vi "Delay Generator SG08p.vi"() -> ()   [LabVIEW 2009, in "POLARIS BME DG.lvlib"]
uses:
  POLARIS BME DG.lvlib
  SubVI/Settings G08.ctl
  <vilib>/Utility/error.llb/DialogType.ctl
panel:
  in  "Settings":T1={"Channel A"={"Delay (µs)"=0.013000000000000001, "Pulse Width (µs)"=0.019, "Output Modulo"=1, "Output Offset"=0, "Go Signal"=16, "Polarity"=TRUE, "Terminate"=FALSE}, "Channel B"={"Delay (µs)"=0.032, "Pulse Width (µs)"=0.019, "Output Modulo"=1, "Output Offset"=0, "Go Signal"=16, "Polarity"=TRUE, "Terminate"=FALSE}, "Channel C"={"Delay (µs)"=0.0, "Pulse Width (µs)"=0.01, "Output Modulo"=1, "Output Offset"=0, "Go Signal"=16, "Polarity"=TRUE, "Terminate"=FALSE}, "Channel D"={"Delay (µs)"=0.01, "Pulse Width (µs)"=0.01, "Output Modulo"=1, "Output Offset"=0, "Go Signal"=16, "Polarity"=TRUE, "Terminate"=FALSE}, "Channel E"={"Delay (µs)"=0.0, "Pulse Width (µs)"=0.01, "Output Modulo"=1, "Output Offset"=0, "Go Signal"=16, "Polarity"=TRUE, "Terminate"=FALSE, "Disconnect"=FALSE, "Onto MsBus"=FALSE, "Input Positive"=TRUE}, "Channel F"={"Delay (µs)"=0.0, "Pulse Width (µs)"=0.01, "Output Modulo"=1, "Output Offset"=0, "Go Signal"=16, "Polarity"=TRUE, "Terminate"=FALSE, "Disconnect"=FALSE, "Onto MsBus"=FALSE, "Input Positive"=TRUE}, "Clock Enable"=TRUE, "Ocillator Divider"=2, "Trigger Divider"=1, "Trigger Multiplier"=4, "Clock Source"=3, "Trigger Terminate"=TRUE, "Gate Terminate"=TRUE, "Trigger Level"=0.2, "Gate Level"=0.0, "Gate Delay (µs)"=-1.0, "MS Bus"=1, "Internal Clock (µs)"=0.0083333, "Stop Trigger"=1, "Gate Divider"=0, "Force Trigger (µs)"=-1.0, "Step Back Time (µs)"=-1.0, "Burst Counter"=1, "Positive Gate"=TRUE, "Trigger Source"=TRUE, "Gate Type"=TRUE, "Synchronize Gate"=FALSE, "Trigger Slope"=TRUE, "Stop on Preset"=FALSE, "Reset When Done"=TRUE, "Trigger Enable"=TRUE, "Gate AB"=0, "Gate CD"=0, "Gate EF"=0} {"Gate EF" items=["Normal"=0, "EF_OR"=1048576, "EF_AND"=2097152, "EF_XOR"=3145728]; "Gate CD" items=["Normal"=0, "CD_OR"=262144, "CD_AND"=524288, "CD_XOR"=786432]; "Gate AB" items=["Normal"=0, "AB_OR"=65536, "AB_AND"=131072, "AB_XOR"=196608]; "Step Back Time (µs)" min=-1.0 format="%.6f"; "Force Trigger (µs)" min=-1.0 format="%.6f"; "Gate Delay (µs)" min=-1.0 format="%.6f"; "Internal Clock (µs)" min=0.0 format="%.6f"; "MS Bus" format="%04x" items=["Local Primary"=1, "Local Secondary"=2, "Local Force"=4, "Resynchronize"=8, "Master Primary"=16, "Master Secondary"=32, "Master Force"=64, "System Clock"=128, "Delay Clock"=256, "Inhibit Local"=512, "Start Local"=1024, "Start Bus"=2048, "Step Back Local"=4096, "Step Back Bus"=8192, "Enable From E"=65536, "Enable From F"=131072, "Enable From Bus"=262144]; "Gate Level" min=-2.5 max=2.5 format="%.3g"; "Trigger Level" min=-2.5 max=2.5 format="%.3f"; "Clock Source" items=["Internal Oscillator"=1, "External Trigger"=2, "Trigger & Oscillator"=3, "Master Slave Bus"=4]; "Trigger Multiplier" min=1; "Trigger Divider" min=1; "Ocillator Divider" min=1; "Channel F"."Go Signal" format="%04x" items=["Loc Prim"=1, "Loc Sec"=2, "Loc Force"=4, "Resynch"=8, "Mas Prim"=16, "Mas Sec"=32, "Mas Force"=64, "Sys Clock"=128, "Delay Clock"=256, "Inhibit Local"=512, "Start Local"=1024, "Start Bus"=2048, "Step Back Loc"=4096, "Step Back Bus"=8192, "From E"=65536, "From F"=131072, "From Bus"=262144]; "Channel F"."Pulse Width (µs)" min=0.0 max=8947840.0 format="%.6f"; "Channel F"."Delay (µs)" min=0.0 format="%.6f"; "Channel E"."Go Signal" format="%04x" items=["Loc Prim"=1, "Loc Sec"=2, "Loc Force"=4, "Resynch"=8, "Mas Prim"=16, "Mas Sec"=32, "Mas Force"=64, "Sys Clock"=128, "Delay Clock"=256, "Inhibit Local"=512, "Start Local"=1024, "Start Bus"=2048, "Step Back Loc"=4096, "Step Back Bus"=8192, "From E"=65536, "From F"=131072, "From Bus"=262144]; "Channel E"."Pulse Width (µs)" min=0.0 max=8947840.0 format="%.6f"; "Channel E"."Delay (µs)" min=0.0 format="%.6f"; "Channel D"."Go Signal" format="%04x" items=["Loc Prim"=1, "Loc Sec"=2, "Loc Force"=4, "Resynch"=8, "Mas Prim"=16, "Mas Sec"=32, "Mas Force"=64, "Sys Clock"=128, "Delay Clock"=256, "Inhibit Local"=512, "Start Local"=1024, "Start Bus"=2048, "Step Back Loc"=4096, "Step Back Bus"=8192, "From E"=65536, "From F"=131072, "From Bus"=262144]; "Channel D"."Pulse Width (µs)" min=0.0 max=8947840.0 format="%.6f"; "Channel D"."Delay (µs)" min=0.0 format="%.6f"; "Channel C"."Go Signal" format="%04x" items=["Loc Prim"=1, "Loc Sec"=2, "Loc Force"=4, "Resynch"=8, "Mas Prim"=16, "Mas Sec"=32, "Mas Force"=64, "Sys Clock"=128, "Delay Clock"=256, "Inhibit Local"=512, "Start Local"=1024, "Start Bus"=2048, "Step Back Loc"=4096, "Step Back Bus"=8192, "From E"=65536, "From F"=131072, "From Bus"=262144]; "Channel C"."Pulse Width (µs)" min=0.0 max=8947840.0 format="%.6f"; "Channel C"."Delay (µs)" min=0.0 format="%.6f"; "Channel B"."Go Signal" format="%04x" items=["Loc Prim"=1, "Loc Sec"=2, "Loc Force"=4, "Resynch"=8, "Mas Prim"=16, "Mas Sec"=32, "Mas Force"=64, "Sys Clock"=128, "Delay Clock"=256, "Inhibit Local"=512, "Start Local"=1024, "Start Bus"=2048, "Step Back Loc"=4096, "Step Back Bus"=8192, "From E"=65536, "From F"=131072, "From Bus"=262144]; "Channel B"."Pulse Width (µs)" min=0.0 max=8947840.0 format="%.6f"; "Channel B"."Delay (µs)" min=0.0 format="%.6f"; "Channel A"."Go Signal" format="%04x" items=["Loc Prim"=1, "Loc Sec"=2, "Loc Force"=4, "Resynch"=8, "Mas Prim"=16, "Mas Sec"=32, "Mas Force"=64, "Sys Clock"=128, "Delay Clock"=256, "Inhibit Local"=512, "Start Local"=1024, "Start Bus"=2048, "Step Back Loc"=4096, "Step Back Bus"=8192, "From E"=65536, "From F"=131072, "From Bus"=262144]; "Channel A"."Pulse Width (µs)" min=0.0 max=8947840.0 format="%.6f"; "Channel A"."Delay (µs)" min=0.0 format="%.6f"}
  in  "Exit":bool
  # "NOTICE -- YOU MUST LEAVE THIS NOTICE IN PLACE.  PER THE TERMS OF THE LICENSE BELOW, YOU MAY SUBLICENSE THIS SOFTWARE \nIN ANY WAY THAT DOES NOT CONFLICT WITH THIS LICENSE.\n\n### BSD License (http://www.opensource.org/licenses/bsd-license.php) Begin ###\n \nCopyright (c) 2011, Applied Energetics, http://www.appliedenergetics.com,\n                               Richard Schwerdtfeger, <rschwerdtfeger@appliedenergetics.com>\n\nAll rights reserved.\n\nRedistribution and use in source and binary forms, with or without modification, are permitted provided that the \nfollowing conditions are met:\n\n    * Redistributions of source code must retain the above copyright notice, this list of conditions and the following disclaimer.\n    * Redistributions in binary form must reproduce the above copyright notice, this list of conditions and the following disclaimer \n       in the documentation and/or other materials provided with the distribution.\n    * Neither the name of Richard Schwerdtfeger, Applied Energetics, Inc., nor the names of its contributors may be used to \n       endorse or promote products derived from this software without specific prior written permission.\n\nTHIS SOFTWARE IS PROVIDED BY THE COPYRIGHT HOLDERS AND CONTRIBUTORS \"AS IS\" AND ANY EXPRESS OR IMPLIED WARRANTIES, \nINCLUDING, BUT NOT LIMITED TO, THE IMPLIED WARRANTIES OF MERCHANTABILITY AND FITNESS FOR A PARTICULAR PURPOSE ARE \nDISCLAIMED. IN NO EVENT SHALL THE COPYRIGHT OWNER OR CONTRIBUTORS BE LIABLE FOR ANY DIRECT, INDIRECT, INCIDENTAL,\n SPECIAL, EXEMPLARY, OR CONSEQUENTIAL DAMAGES (INCLUDING, BUT NOT LIMITED TO, PROCUREMENT OF SUBSTITUTE GOODS OR \nSERVICES; LOSS OF USE, DATA, OR PROFITS; OR BUSINESS INTERRUPTION) HOWEVER CAUSED AND ON ANY THEORY OF LIABILITY, \nWHETHER IN CONTRACT, STRICT LIABILITY, OR TORT (INCLUDING NEGLIGENCE OR OTHERWISE) ARISING IN ANY WAY OUT OF THE USE \nOF THIS SOFTWARE, EVEN IF ADVISED OF THE POSSIBILITY OF SUCH DAMAGE.\n\n### BSD License End ###"
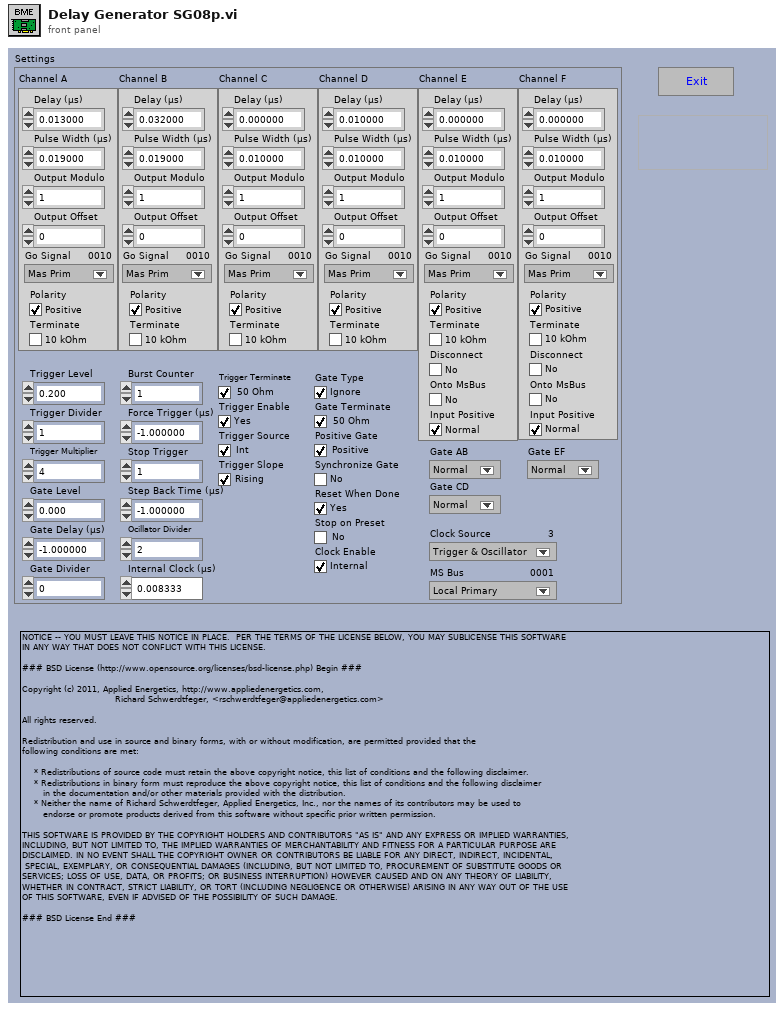
[diagram p1: front panel]
types:
  T1 = typedef "POLARIS BME DG.lvlib/Settings G08.ctl" = cluster{"Channel A":cluster{"Delay (µs)":dbl, "Pulse Width (µs)":dbl, "Output Modulo":u32, "Output Offset":u32, "Go Signal":u32, "Polarity":bool, "Terminate":bool}, "Channel B":cluster{"Delay (µs)":dbl, "Pulse Width (µs)":dbl, "Output Modulo":u32, "Output Offset":u32, "Go Signal":u32, "Polarity":bool, "Terminate":bool}, "Channel C":cluster{"Delay (µs)":dbl, "Pulse Width (µs)":dbl, "Output Modulo":u32, "Output Offset":u32, "Go Signal":u32, "Polarity":bool, "Terminate":bool}, "Channel D":cluster{"Delay (µs)":dbl, "Pulse Width (µs)":dbl, "Output Modulo":u32, "Output Offset":u32, "Go Signal":u32, "Polarity":bool, "Terminate":bool}, "Channel E":cluster{"Delay (µs)":dbl, "Pulse Width (µs)":dbl, "Output Modulo":u32, "Output Offset":u32, "Go Signal":u32, "Polarity":bool, "Terminate":bool, "Disconnect":bool, "Onto MsBus":bool, "Input Positive":bool}, "Channel F":cluster{"Delay (µs)":dbl, "Pulse Width (µs)":dbl, "Output Modulo":u32, "Output Offset":u32, "Go Signal":u32, "Polarity":bool, "Terminate":bool, "Disconnect":bool, "Onto MsBus":bool, "Input Positive":bool}, "Clock Enable":bool, "Ocillator Divider":u32, "Trigger Divider":u32, "Trigger Multiplier":u32, "Clock Source":u32, "Trigger Terminate":bool, "Gate Terminate":bool, "Trigger Level":dbl, "Gate Level":dbl, "Gate Delay (µs)":dbl, "MS Bus":u32, "Internal Clock (µs)":dbl, "Stop Trigger":u32, "Gate Divider":u32, "Force Trigger (µs)":dbl, "Step Back Time (µs)":dbl, "Burst Counter":u32, "Positive Gate":bool, "Trigger Source":bool, "Gate Type":bool, "Synchronize Gate":bool, "Trigger Slope":bool, "Stop on Preset":bool, "Reset When Done":bool, "Trigger Enable":bool, "Gate AB":u32, "Gate CD":u32, "Gate EF":u32}
  T2 = typedef "DialogType.ctl" = u16
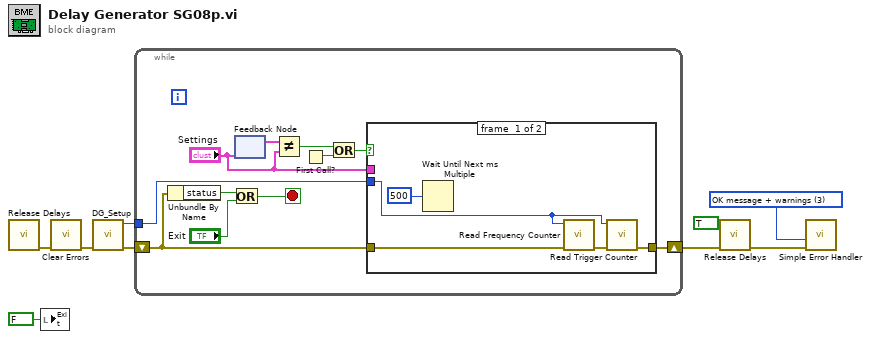
[diagram p0: block diagram]
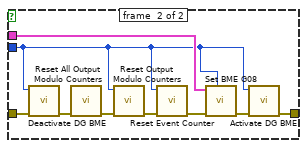
[diagram p2: hidden frame]
diagram:
  w2 = T2 3 items=["no dialog", "OK message", "continue or stop message", "OK message + warnings", "continue/stop + warnings"] ("type of dialog (OK msg:1)")
  n1 = call "Release Delays.vi"() -> ("error out"=w8:errorcluster)  [unwired: 2 in, 9 out]
  n2 = local write "Exit"(FALSE ("Stop")) -> ()
  n3 = call <vilib>:"Clear Errors.vi"("error in (no error)"=w8) -> ("error out"=w7:errorcluster)  [unwired: 6 out]
  n4 = call "DG_Setup.vi"("error in (no error)"=w7) -> ("error out"=w9:errorcluster, "DG Number"=w6:i32)  [unwired: 2 in, 7 out]
  n5 = while {
    shift-right: [w17] -> w5
    shift-left: w9 -> [w15]
    tunnel: w6 -> [w16]
    stop <- w20 stop-if-true
    n6 = Unbundle By Name(w15) -> ("status"=w18:bool)
    n7 = Or(x=w18, y="Exit") -> (x .or. y?=w20:bool)
    n8 = feedback #1("Settings") -> (w13:T1)
    n9 = Not Equal?(x=w13, y="Settings") -> (x != y?=w14:bool)
    n10 = First Call?() -> (First Call?: T/F=w12:bool)
    n11 = Or(x=w14, y=w12) -> (x .or. y?=w10:bool)
    n12 = case shown="True" w10 {
      tunnel: [w22 w28] -> w17
      tunnel: w15 -> [w24 w29]
      tunnel: "Settings" -> [_ w30]
      tunnel: w16 -> [w21 w27]
      frame #0 {
        n13 = Wait Until Next ms Multiple(millisecond multiple=u32 500) -> ()  [unwired: 1 out]
        n14 = call "Read Frequency Counter.vi"("error in (no error)"=w24, "DG_Number"=w21) -> ("error out"=w23:errorcluster)  [unwired: 1 in, 8 out]
        n15 = call "Read Trigger Counter.vi"("error in (no error)"=w23, "DG Number"=w21) -> ("error out"=w22:errorcluster)  [unwired: 9 out]
      }
      frame #1 {
        n16 = call "Deactivate DG BME.vi"("error in (no error)"=w29, "DG Number"=w27) -> ("error out"=w34:errorcluster)  [unwired: 9 out]
        n17 = call "Reset All Output Modulo Counters.vi"("error in (no error)"=w34) -> ("error out"=w33:errorcluster)  [unwired: 10 out]
        n18 = call "Reset Output Modulo Counters.vi"("error in (no error)"=w33, "DG Number"=w27) -> ("error out"=w32:errorcluster)  [unwired: 9 out]
        n19 = call "Reset Event Counter.vi"("error in (no error)"=w32, "DG Number"=w27) -> ("error out"=w31:errorcluster)  [unwired: 9 out]
        n20 = call "Set BME G08.vi"("DG Number"=w27, "error in (no error)"=w31, "Settings"=w30) -> ("error out"=w26:errorcluster)  [unwired: 8 out]
        n21 = call "Activate DG BME.vi"("error in (no error)"=w26, "DG Number"=w27) -> ("error out"=w28:errorcluster)  [unwired: 9 out]
      }
    }
  }
  n22 = call "Release Delays.vi"("error in (no error)"=w5, "Release"=TRUE) -> ("error out"=w1:errorcluster)  [unwired: 9 out]
  n23 = call <vilib>:"Simple Error Handler.vi"("type of dialog (OK msg:1)"=w2, "error in (no error)"=w1) -> ()  [unwired: 8 out]
